vi "Clear change list.vi"(8 "error in (no error)":errorcluster, 11 "Fiber Auto Collimation state data in":refnum<class "Fiber Auto Collimation state data.lvclass">) -> (0 "error out":errorcluster, 3 "Fiber Auto Collimation state data out":refnum<class "Fiber Auto Collimation state data.lvclass">)   [LabVIEW 2018, in "Fiber Auto Collimation state data.lvclass"]
doc: "Clears the \"data changed\" list. Should usually only ever be called right after an event to send the data to all listeners has been activated."
uses:
  Fiber Auto Collimation state data.lvclass
  Tracked state data.ctl
  Fiber Auto Collimation state data.lvclass/Fiber Auto Collimation state data.ctl
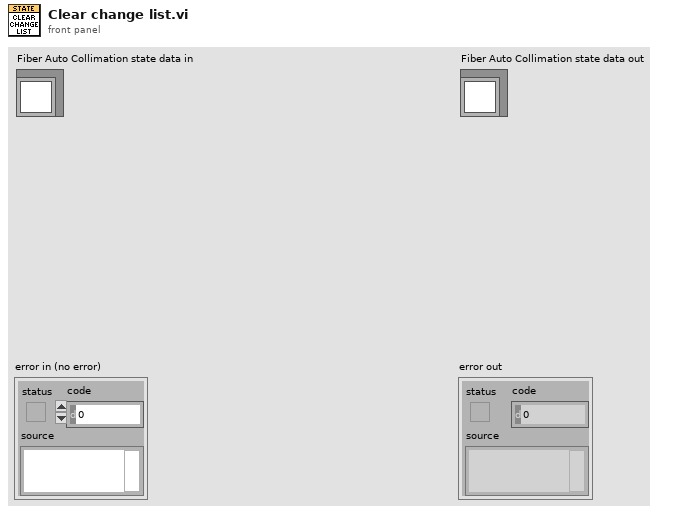
[diagram p1: front panel]
types:
  T1 = typedef "Fiber Auto Collimation state data.lvclass/Tracked state data.ctl" = enum16{"No update", "Permission level", "Username", "Test running", "DUT Serial", "Test status", "MOM Lot", "Loaded test recipe", "Model case running", "Station status", "BV data", "Defect Identify data", "Axis Position data", "Fiber Ass PN", "Operator", "RunTime", "VBAI", "Steps Cycle Time"}
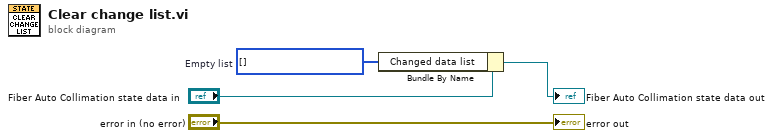
[diagram p0: block diagram]
diagram:
  w1 = T1[] [] items=["No update", "Permission level", "Username", "Test running", "DUT Serial", "Test status", "MOM Lot", "Loaded test recipe", "Model case running", "Station status", "BV data", "Defect Identify data", "Axis Position data", "Fiber Ass PN", "Operator", "RunTime", "VBAI", "Steps Cycle Time"]  # Empty list
  n1 = Bundle By Name(cluster="Fiber Auto Collimation state data in", "Changed data list"=w1) -> (→"Fiber Auto Collimation state data out":refnum<class "Fiber Auto Collimation state data.lvclass">)
  "error out" <- "error in (no error)"
